vi "Capture DAQ Timestamp.vi"(0 "DaqData dCVT":T1, 1 "timestamp in":dbl, 3 "error in (no error)":errorcluster, 4 "AI TaskName":string) -> (7 "DaqData dCVT out":T1, 8 "Timestamp":dbl, 10 "error out":errorcluster)   [LabVIEW 2017, in "DAQ.lvclass"]
doc: "Developed by Kevin Thompson\nkevin@thompsonengineering.net\n\nCopyright 2018-2020\nThompson Engineering, LLC\nAI scan timestamp is stored with IOName \"%sScanTS\" in DAQ Data Dict\n(%s = ['AI' | 'DI'])"
uses:
  DAQ.lvclass
  <vilib>/TELLC/Dynamic CVT API/TD Dynamic CVT DVR--ref.ctl
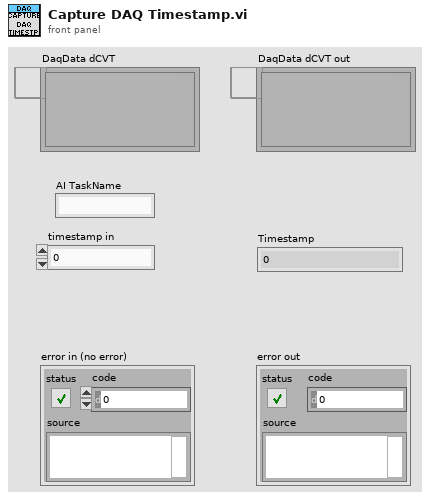
[diagram p1: front panel]
types:
  T1 = typedef "TD Dynamic CVT DVR--ref.ctl" = refnum<data-value>
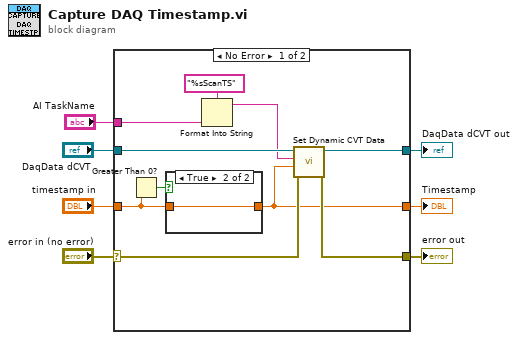
[diagram p0: block diagram]
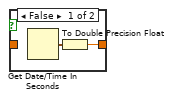
[diagram p2: hidden frame]
diagram:
  n1 = case shown="No Error" "error in (no error)" {
    selector: "error in (no error)" -> [w14 w21]
    tunnel: [w17 w21] -> w7
    tunnel: [w16 w22] -> w6
    tunnel: "DaqData dCVT" -> [w15 w22]
    tunnel: [w13 _] -> w3
    tunnel: "timestamp in" -> [w11 _]
    tunnel: "AI TaskName" -> [w10 _]
    frame No Error {
      n2 = Greater Than 0?(x=w11) -> (x > 0?=w12:bool)
      n3 = case shown="True" w12 {
        tunnel: [w18 w20] -> w13
        tunnel: w11 -> [_ w20]
        frame False {
          n4 = Get Date/Time In Seconds() -> (seconds since 1Jan1904=w19:timestamp)
          n5 = To Double Precision Float(number=w19) -> (double precision float=w18:dbl)
        }
        frame True {
        }
      }
      n6 = Format Into String(format string="%sScanTS" ("initial string"), w10) -> (resulting string=w8:string)  [unwired: 2 in, 1 out]
      n7 = call <vilib>:"Set Dynamic CVT Data.vi"("error in (no error)"=w14, "value"=w13, "DataName"=w8, "dCVT DVR"=w15) -> ("error out"=w17:errorcluster, "dCVT DVR out"=w16:T1)  [unwired: 5 in, 1 out]
    }
    frame Error {
    }
  }
  "error out" <- w7
  "DaqData dCVT out" <- w6
  "Timestamp" <- w3
